vi "Read Second Dichotomie.vi"(11 "Collision in":refnum<class "Collision.lvclass">) -> (2 "Second Dichotomie":i32)   [LabVIEW 2024, in "Collision.lvclass"]
doc: "MIT Licence\nCopyright (c) 2024 David Grollier"
uses:
  Collision.lvclass
  Collision.lvclass/Collision.ctl
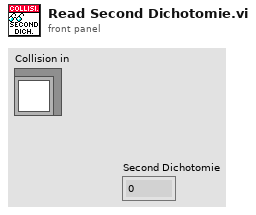
[diagram p1: front panel]
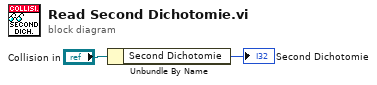
[diagram p0: block diagram]
diagram:
  n1 = Unbundle By Name("Collision in") -> ("Second Dichotomie"=→"Second Dichotomie":i32)
